vi "Subvi FIFO OUT b.vi"(0 "FIFO OUT debug":bool, 4 "number 8":u8, 5 "number 1":u8, 6 "number 7":u8, 7 "number 2":u8, 8 "number 6":u8, 9 "number 5":u8, 10 "number 4":u8, 11 "number 3":u8) -> (1 "Push FIFO OUT mon":bool)   [LabVIEW 2017]
uses:
  GV FIFO OUT gate.vi
  GV gated pixel clock change.vi
  <vilib>/rvi/Emulation/niFpgaEmulationIsFPGAContextNoSignature.vi
  <vilib>/rvi/Emulation/niFpgaSctlEmulationGetInTimedLoop.vi
  <vilib>/rvi/errors/niFpgaSetErrorForExecOnDevCompSimple.vi
  <vilib>/rvi/eio/common/nirviEmuReportErrorAndStop.vi
  <vilib>/rvi/DataTransferAndStorage/Container/Common/niFpgaContainerGetUniqueNameForEmu.vi
  <vilib>/rvi/FIFO/Fifo_Resource/nirvififoEmulationSetSize.vi
  <vilib>/rvi/FIFO/Fifo_Resource/nirviFifoEmulationQueueMgr.vi
  <instcachedir>/0/nirviFifoEmulationQueueMgr_E5CAEC123FF24DC58D834DCA3CDAA9B5.lvgen/nirviFifoEmulationQueueMgr_E5CAEC123FF24DC58D834DCA3CDAA9B5_001.vi
  <vilib>/Utility/error.llb/Clear Errors.vi
  <vilib>/rvi/FIFO/Fifo_Resource/nirvififoEmulationCreateLock.vi
  <vilib>/rvi/Emulation/niFpgaProcessEmulError.vi
  <vilib>/rvi/FIFO/Fifo_Resource/nirvififoEmulationObtainLock.vi
  <vilib>/rvi/FIFO/Fifo_Resource/nirvififoEmulationReleaseLock.vi
  <vilib>/rvi/occurrence/nirviWaitOnOccurrenceBase.vi
  <vilib>/rvi/errors/nirviReportUnexpectedCaseInternalError.vi
  <vilib>/rvi/errors/nirviReportUnexpectedCaseInternalError (U32).vi
  <vilib>/rvi/interface/RandomDataEmulation/niFpgaRandomDataHandleErrors.vi
  <vilib>/rvi/FIFO/Fifo_Resource/nirvififoEmulationDetermineInputValidOut.vi
  <vilib>/rvi/DataTransferAndStorage/Container/XNode/niFpgaContainer.xnode
  <vilib>/rvi/FIFO/Fifo_Resource/nirvififoEmulationRead.vi
  <vilib>/rvi/interface/RandomDataEmulation/nirviRandomDataFpgaReadWriteTemplate.vi
  <vilib>/rvi/FIFO/Fifo_Resource/nirvififoEmulationWrite.vi
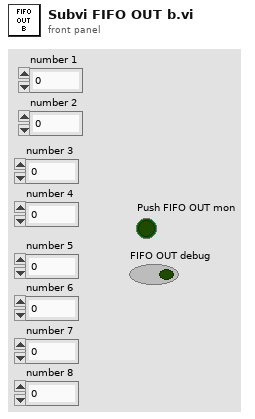
[diagram p1: front panel]
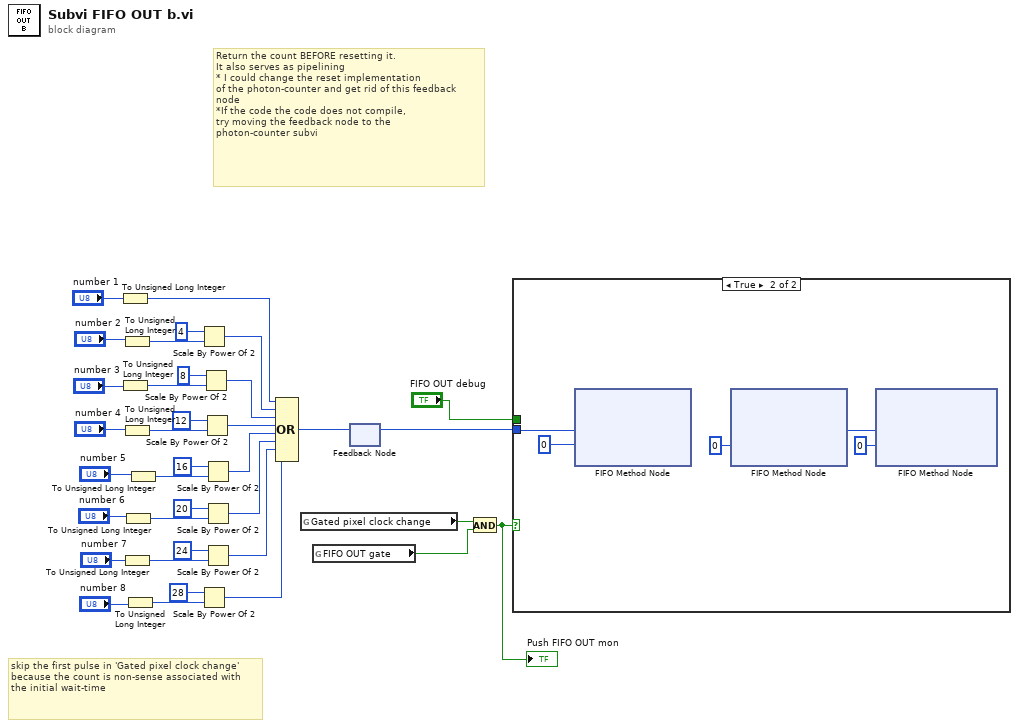
[diagram p0: block diagram]
diagram:
  # "Return the count BEFORE resetting it.\nIt also serves as pipelining\n* I could change the reset implementation\nof the photon-counter and get rid of this feedback node\n*If the code the code does not compile,\ntry moving the feedback node to the\nphoton-counter subvi"
  # "skip the first pulse in 'Gated pixel clock change'\nbecause the count is non-sense associated with\nthe initial wait-time"
  n1 = To Unsigned Long Integer(number="number 1") -> (unsigned 32bit integer=w21:u32)
  n2 = To Unsigned Long Integer(number="number 3") -> (unsigned 32bit integer=w19:u32)
  n3 = To Unsigned Long Integer(number="number 2") -> (unsigned 32bit integer=w20:u32)
  n4 = To Unsigned Long Integer(number="number 4") -> (unsigned 32bit integer=w18:u32)
  n5 = To Unsigned Long Integer(number="number 7") -> (unsigned 32bit integer=w15:u32)
  n6 = To Unsigned Long Integer(number="number 6") -> (unsigned 32bit integer=w16:u32)
  n7 = To Unsigned Long Integer(number="number 8") -> (unsigned 32bit integer=w14:u32)
  n8 = To Unsigned Long Integer(number="number 5") -> (unsigned 32bit integer=w17:u32)
  n9 = Scale By Power Of 2(n=i16 4, x=w20) -> (x*2^n=w28:u32)
  n10 = Scale By Power Of 2(n=i16 28, x=w14) -> (x*2^n=w22:u32)
  n11 = Scale By Power Of 2(n=i16 8, x=w19) -> (x*2^n=w27:u32)
  n12 = Scale By Power Of 2(n=i16 12, x=w18) -> (x*2^n=w26:u32)
  n13 = Scale By Power Of 2(n=i16 16, x=w17) -> (x*2^n=w25:u32)
  n14 = Scale By Power Of 2(n=i16 20, x=w16) -> (x*2^n=w24:u32)
  n15 = Scale By Power Of 2(n=i16 24, x=w15) -> (x*2^n=w23:u32)
  n16 = Compound Arithmetic op=OR(w21, w28, w27, w26, w25, w24, w23, w22) -> (w4:u32)
  n17 = global read "GV gated pixel clock change.vi" "Gated pixel clock change"() -> (w5:bool)
  n18 = global read "GV FIFO OUT gate.vi" "FIFO OUT gate"() -> (w2:bool)
  n19 = feedback-in #1(w4) -> ()
  n20 = feedback #1() -> (w3:u32)  [unwired: 1 in]
  n21 = And(x=w5, y=w2) -> (x .and. y?=w1:bool)
  "Push FIFO OUT mon" <- w1
  n22 = case shown="True" w1 {
    tunnel: "FIFO OUT debug" -> [_ _]
    tunnel: w3 -> [_ w40]
    frame False {
    }
    frame True {
      n23 = xnode ("FIFO Method Node")("Element"=w40, "Timeout"=0) -> ()  [unwired: 1 in, 2 out]
      n24 = xnode ("FIFO Method Node")("Timeout"=0) -> ("Element"=w39:u32)  [unwired: 1 in, 2 out]
      n25 = xnode ("FIFO Method Node")("Element"=w39, "Timeout"=0) -> ()  [unwired: 1 in, 2 out]
    }
  }
